vi "setParent.vi"(0 "reference":refnum<class "AbstractNode.lvclass">, 1 "node":refnum<class "AbstractNode.lvclass">, 5 "error in (no error)":errorcluster) -> (14 "reference out":refnum<class "AbstractNode.lvclass">, 19 "error out":errorcluster)   [LabVIEW 2016, in "AbstractNode.lvclass"]
doc: "public void setParent(Node node)"
uses:
  <resource>/Framework/Providers/Open_GDS/UML/AbstractNode_class/AbstractNode.lvclass
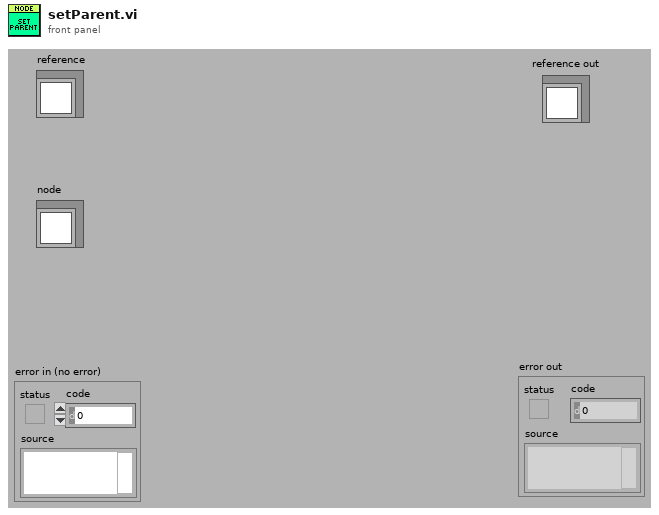
[diagram p1: front panel]
types:
  T1 = typedef "AbstractNode.lvclass/ObjectAttributes.ctl" = cluster{"parent":refnum<class "AbstractNode.lvclass">, "children":refnum<class "AbstractNode.lvclass">[], "Hidden":bool}
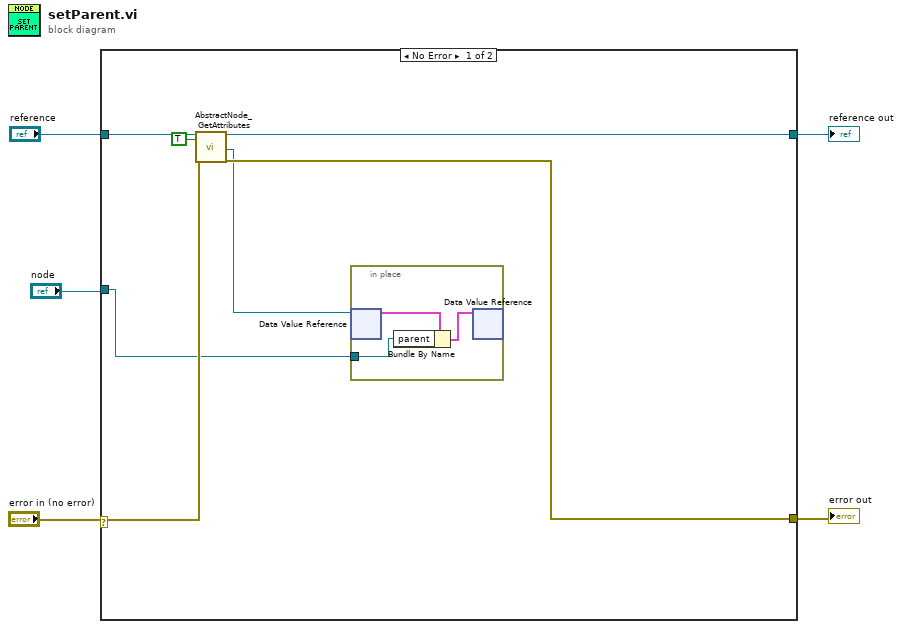
[diagram p0: block diagram]
diagram:
  n1 = case shown="No Error" "error in (no error)" {
    selector: "error in (no error)" -> [w9 w16]
    tunnel: "reference" -> [w12 w17]
    tunnel: [w11 w16] -> w4
    tunnel: [w10 w17] -> w3
    tunnel: "node" -> [w6 _]
    frame No Error {
      n2 = call <resource>:"AbstractNode_GetAttributes.vi"("reference in"=w12, "OnlyGetDvrReference(False)"=TRUE, "error in (no error)"=w9) -> ("reference out"=w10:refnum<class "AbstractNode.lvclass">, "DataRef"=w7:refnum<data-value>, "error out"=w11:errorcluster)  [unwired: 13 in, 1 out]
      n3 = in-place {
        in-place-border: w6 -> [w14]
        n4 = in-place-dvr #1(w7) -> (w15:T1)  [unwired: 1 out]
        n5 = Bundle By Name(cluster=w15, "parent"=w14) -> (w13:T1)
        n6 = in-place-dvr #1(w13) -> ()  [unwired: 2 out]
      }
    }
    frame Error {
    }
  }
  "reference out" <- w3
  "error out" <- w4
